vi "Get nElements.vi"(11 "Priority Queue in":refnum<class "NI_Robotics_Priority Queue.lvclass">) -> (2 "nElements":i32, 3 "Priority Queue out":refnum<class "NI_Robotics_Priority Queue.lvclass">)   [LabVIEW 2017, in "NI_Robotics_Priority Queue.lvclass"]
uses:
  <vilib>/robotics/Navigation/shared/Priority Queue/NI_Robotics_Priority Queue.lvclass
  <vilib>/robotics/Navigation/shared/Priority Queue/NI_Robotics_Priority Queue.lvclass/NI_Robotics_Priority Queue.ctl
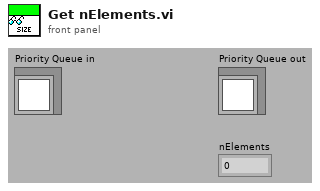
[diagram p1: front panel]
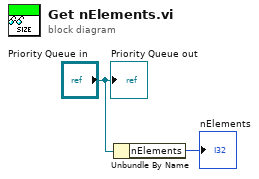
[diagram p0: block diagram]
diagram:
  n1 = Unbundle By Name("Priority Queue in") -> ("nElements"=→"nElements":i32)
  "Priority Queue out" <- "Priority Queue in"
